vi "CANopen_SDOread.vi"() -> ()   [LabVIEW 2013]
uses:
  <vilib>/CANopenLib/CANOPEN.llb/CANopen BaudRate.ctl
  <vilib>/Platform/TimedLoop/XDataNode/timing_clust.ctl
  <vilib>/Platform/TimedLoop/XDataNode/nitl_modes.ctl
  <vilib>/Platform/TimedLoop/XDataNode/wakeup.ctl
  <vilib>/CANopenLib/CANOPEN.llb/CANopen Interface Create.vi
  <vilib>/CANopenLib/CANOPEN.llb/CANopen SDO Create.vi
  <vilib>/CANopenLib/CANOPEN.llb/CANopen SDO Close.vi
  <vilib>/CANopenLib/CANOPEN.llb/CANopen Interface Close.vi
  <vilib>/CANopenLib/CANOPEN.llb/CANopen SDO Read [STR].vi
  <vilib>/Platform/TimedLoop/XDataNode/XDataNode.xnode
  <vilib>/Platform/TimedLoop/XDataNode/XDNodeRunTimeDep.lvlib
panel:
  out "description":string
  out "string data":string
  out "error out 2":errorcluster
  out "Completion Code 2":u32 format="%.0x"
  in  "Subindex 2":u8=2 format="%.0x"
  in  "Object Index 2":u16=6144 format="%.0x"
  in  "?":bool
  in  "Node-ID":u8=1 min=1 max=127 step=1
  in  "error in":errorcluster
  out "error out":errorcluster
  in  "Baud Rate":T1=2 items=["1 Mbit/s"=0, "800 kbit/s"=1, "500 kbit/s"=2, "250 kbit/s"=3, "125 kbit/s"=4, "50 kbit/s"=6, "20 kbit/s"=7, "10 kbit/s"=8]
  in  "CANopen Interface":u32(ring) items=["CANopen01", "CANopen02", "CANopen03", "CANopen04", "CANopen05", "CANopen06", "CANopen07", "CANopen08", "CANopen09", "CANopen10", "CANopen11", "CANopen12", "CANopen13", "CANopen14", "CANopen15", "CANopen16", "CANopen17", "CANopen18", "CANopen19", "CANopen20", "CANopen21", "CANopen22", "CANopen23", "CANopen24", "CANopen25", "CANopen26", "CANopen27", "CANopen28", "CANopen29", "CANopen30", "CANopen31", "CANopen32"]
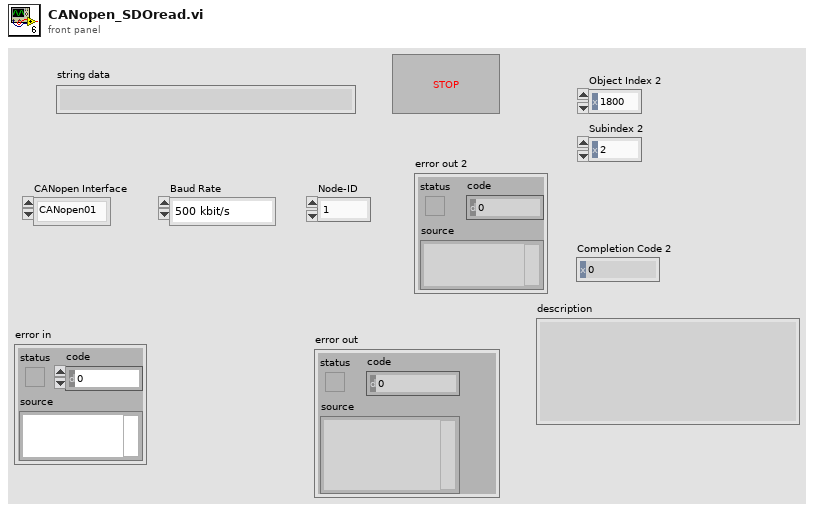
[diagram p1: front panel]
types:
  T1 = typedef "CANopen BaudRate.ctl" = u32
  T2 = typedef "XDNodeRunTimeDep.lvlib/timing_clust.ctl" = cluster{"Expected End [f-1]":u64, "Actual End [f-1]":u64, "Finished Late? [f-1]":bool, "Expected End [i-1]":u64, "Actual End [i-1]":u64, "Finished Late? [i-1]":bool, "Expected Start [i]":u64, "Actual Start [i]":u64, "Expected Start [f]":u64, "Actual Start [f]":u64, "Source Name":string, "Structure Name":string, "Period":i64, "Deadline":i64, "Offset":i64, "Start":i64, "Priority":i32, "Timeout":i32, "Mode":T3, "Wakeup Reason":T4, "Error":errorcluster, "Source Type":string, "Secondary Source Type":string, "Global End Time":u64, "Global Start Time":u64, "Frame Duration":u64, "Iteration Duration":u64, "Assigned CPU":i32, "I/O Scan Engine Mode":u32}
  T3 = typedef "XDNodeRunTimeDep.lvlib/nitl_modes.ctl" = enum32{"No Change", "Process missed periods, maintain original phase", "Discard missed periods, maintain original phase", "Process missed periods, ignore original phase", "Discard missed periods, ignore original phase"}
  T4 = typedef "XDNodeRunTimeDep.lvlib/wakeup.ctl" = enum32{"Normal", "Aborted", "Asynchronous wakeup", "Timing source error", "Timed loop error", "Timeout"}
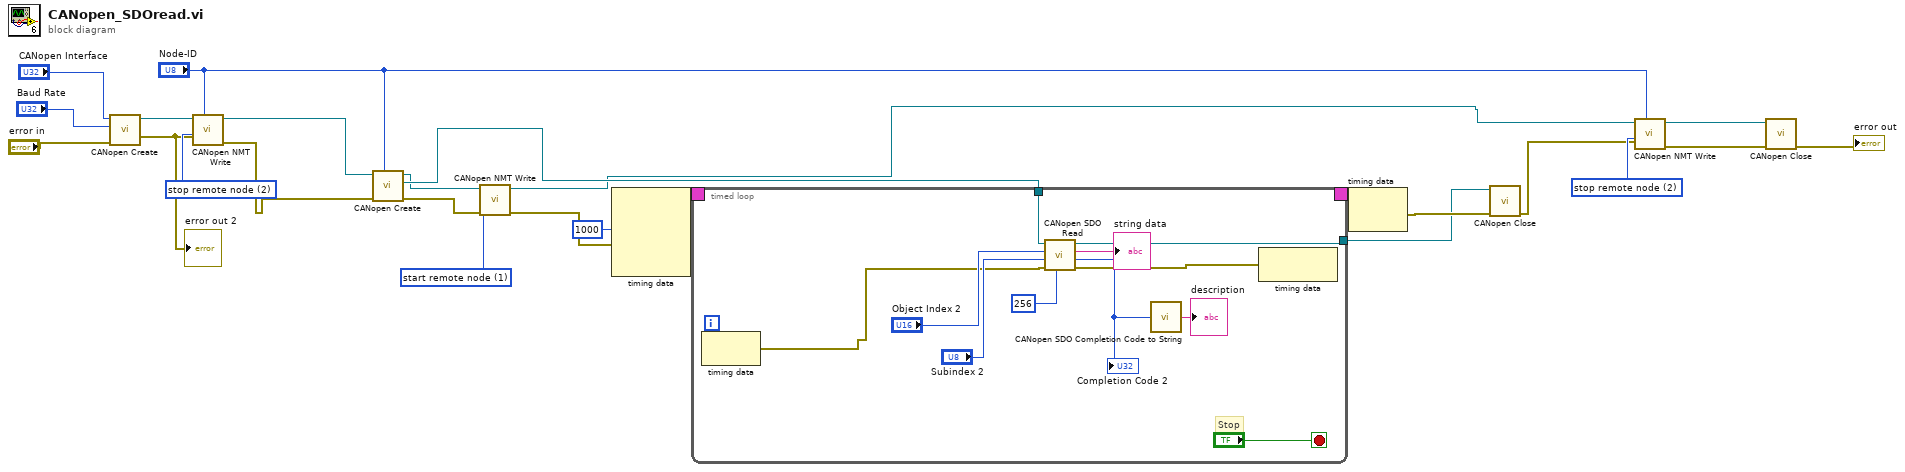
[diagram p0: block diagram]
diagram:
  w2 = u16 1 items=["start remote node"=1, "stop remote node"=2, "enter pre-operational"=128, "reset node"=129, "reset communication"=130] ("command")
  w20 = u16 2 items=["start remote node"=1, "stop remote node"=2, "enter pre-operational"=128, "reset node"=129, "reset communication"=130] ("command")
  w23 = u16 2 items=["start remote node"=1, "stop remote node"=2, "enter pre-operational"=128, "reset node"=129, "reset communication"=130] ("command")
  n1 = call-poly <vilib>:"CANopen Create.vi"("error in (no error)"="error in", "baud rate"="Baud Rate", "interface name"="CANopen Interface") -> ("error out"=w22:errorcluster, "interface object out"=w21:refnum<k20>)  [unwired: 7 in]
  "error out 2" <- w22
  n2 = call <vilib>:"CANopen NMT Write.vi"("node-ID (0)"="Node-ID", "error in (no error)"=w22, "command"=w23, "interface object in"=w21) -> ("error out"=w9:errorcluster, "interface object out"=w10:refnum<k20>)  [unwired: 6 in]
  n3 = call-poly <vilib>:"CANopen Create.vi"("node-ID"="Node-ID", "error in (no error)"=w9, "interface object in"=w10) -> ("error out"=w6:errorcluster, "SDO object out"=w7:refnum<k20>, "interface object out"=w4:refnum<k20>)  [unwired: 6 in]
  n4 = call <vilib>:"CANopen NMT Write.vi"("error in (no error)"=w6, "command"=w2, "interface object in"=w4) -> ("error out"=w5:errorcluster, "interface object out"=w3:refnum<k20>)  [unwired: 7 in]
  n5 = node-c288(i64 1000 ("Periode"), w5) -> (w14:T2)  [unwired: 2 in]
  n6 = timed-loop {
    timing: w14 -> [_]
    timing-out: [_] -> w13
    tunnel: [w31] -> w11
    tunnel: w7 -> [w29]
    stop <- "?" stop-if-true
    # "Stop"
    n7 = node-c288() -> (w30:errorcluster)  [unwired: 1 in]
    n8 = call-poly <vilib>:"CANopen SDO Read.vi"("data size"=u32 256, "error in (no error)"=w30, "object sub-index (0)"="Subindex 2", "object index"="Object Index 2", "SDO object in"=w29) -> ("error out"=w33:errorcluster, "completion code"=w32:u32, "string data"=→"string data":string, "SDO object out"=w31:refnum<k20>)  [unwired: 3 in]
    "Completion Code 2" <- w32
    n9 = call <vilib>:"CANopen SDO Completion Code to String.vi"("SDO completion code"=w32) -> ("description"=→"description":string)
    n10 = node-c288(w33) -> ()  [unwired: 1 out]
  }
  n11 = node-c288(w13) -> (w12:errorcluster)
  n12 = call-poly <vilib>:"CANopen Close.vi"("error in (no error)"=w12, "SDO object in"=w11) -> ("error out"=w18:errorcluster)  [unwired: 9 in]
  n13 = call <vilib>:"CANopen NMT Write.vi"("node-ID (0)"="Node-ID", "error in (no error)"=w18, "command"=w20, "interface object in"=w3) -> ("error out"=w17:errorcluster, "interface object out"=w15:refnum<k20>)  [unwired: 6 in]
  n14 = call-poly <vilib>:"CANopen Close.vi"("error in (no error)"=w17, "interface object in"=w15) -> ("error out"=→"error out":errorcluster)  [unwired: 9 in]
